vi "List Test Node MAC.vi"(8 "error in (no error)":errorcluster, 11 "Create Test Node Model in":refnum<class "Create Test Node Model.lvclass">) -> (0 "error out":errorcluster, 3 "Create Test Node Model out":refnum<class "Create Test Node Model.lvclass">)   [LabVIEW 2013, in "Create Test Node Model.lvlib" / "Create Test Node Model.lvclass"]
uses:
  Create Test Node Model.lvclass
  Create Test Node Model.lvclass/Create Test Node Model.ctl
  <vilib>/ActorFrameworkMVC/View Observer/View Registry/View Registry.lvclass/View Registry.ctl
  Create Test Node Model Messages/Abstract Create Test Node List Msg/Abstract Create Test Node List Msg.lvclass
  <vilib>/ActorFrameworkMVC/View Observer/Data Message/Data Message.lvclass
  <vilib>/ActorFrameworkMVC/View Observer/View Registry/View Registry.lvclass
  Common/ZDAQ/ZDAQ.lvlib
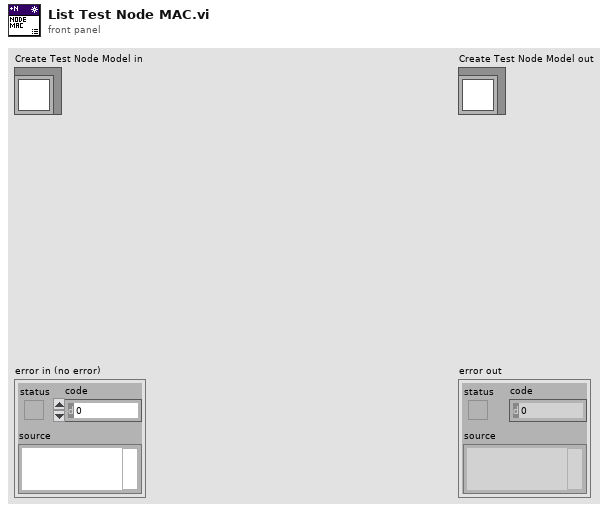
[diagram p1: front panel]
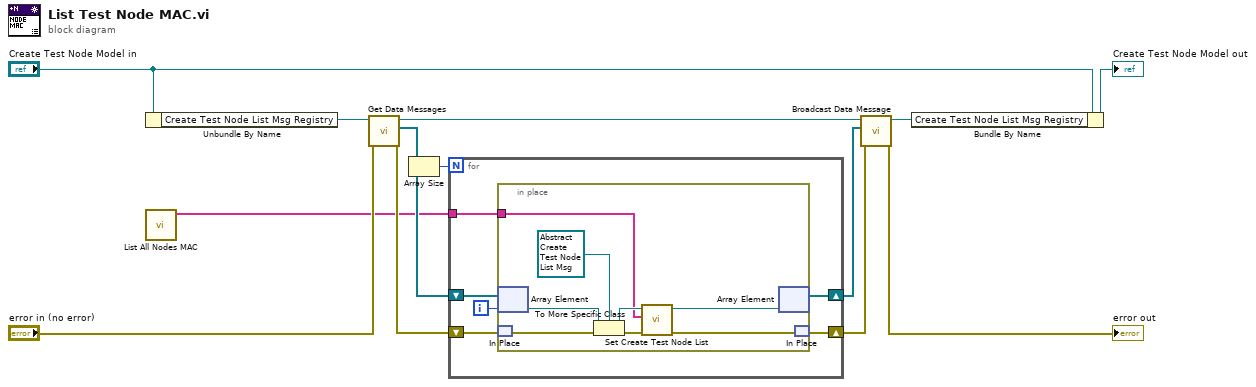
[diagram p0: block diagram]
diagram:
  n1 = Unbundle By Name("Create Test Node Model in") -> ("Create Test Node List Msg Registry"=w13:refnum<class "View Registry.lvclass">)
  n2 = call "List All Nodes MAC.vi"() -> ("Nodes MAC List"=w1:string[])  [unwired: 10 in, 1 out]
  n3 = call <vilib>:"Get Data Messages.vi"("error in (no error)"="error in (no error)", "View Registry in"=w13) -> ("error out"=w9:errorcluster, "Data Messages"=w10:refnum<class "Data Message.lvclass">[], "View Registry out"=w12:refnum<class "View Registry.lvclass">)  [unwired: 7 in]
  n4 = Array Size(array=w10) -> (size(s)=w11:i32)
  n5 = for {
    N: w11 -> [_]
    shift-right: [w18] -> w8
    shift-left: w10 -> [w19]
    shift-right: [w15] -> w7
    shift-left: w9 -> [w17]
    tunnel: w1 -> [w16]
    i -> [w14]
    n6 = in-place {
      in-place-border: w16 -> [w20]
      n7 = in-place-array #1(w19, w14) -> (w25:refnum<class "Data Message.lvclass">)
      n8 = in-place-match #2(w17) -> (w27:errorcluster)
      n9 = To More Specific Class(target class=refnum<class "Abstract Create Test Node List Msg.lvclass"> refnum ("Create Test Node Model.lvlib:Abstract Create Test Node List Msg.lvclass"), reference=w25, error in=w27) -> (specific class reference=w21:refnum<class "Abstract Create Test Node List Msg.lvclass">, error out=w24:errorcluster)
      n10 = call "Set Create Test Node List.vi"("error in (no error)"=w24, "Create Test Node List"=w20, "Abstract Create Test Node List Msg in"=w21) -> ("error out"=w23:errorcluster, "Abstract Create Test Node List Msg out"=w22:refnum<class "Abstract Create Test Node List Msg.lvclass">)  [unwired: 7 in]
      n11 = in-place-array #1(w22) -> (w18:refnum<class "Data Message.lvclass">[])  [unwired: 1 out]
      n12 = in-place-match #2(w23) -> (w15:errorcluster)
    }
  }
  n13 = call <vilib>:"Broadcast Data Message.vi"("error in (no error)"=w7, "Data Messages"=w8, "View Registry in"=w12) -> ("error out"=→"error out":errorcluster, "View Registry out"=w6:refnum<class "View Registry.lvclass">)  [unwired: 7 in]
  n14 = Bundle By Name(cluster="Create Test Node Model in", "Create Test Node List Msg Registry"=w6) -> (→"Create Test Node Model out":refnum<class "Create Test Node Model.lvclass">)
